vi "_getViDocumentationInfo.vi"(8 "error in (no error)":errorcluster, 11 "VI in":refnum<vi>) -> (0 "error out":errorcluster, 1 "Bookmarks":string[][](array[string]), 2 "VI Documentation Info":T1, 3 "VI out":refnum<vi>)   [LabVIEW 2017]
doc: "Returns the documentation information for the specified VI reference."
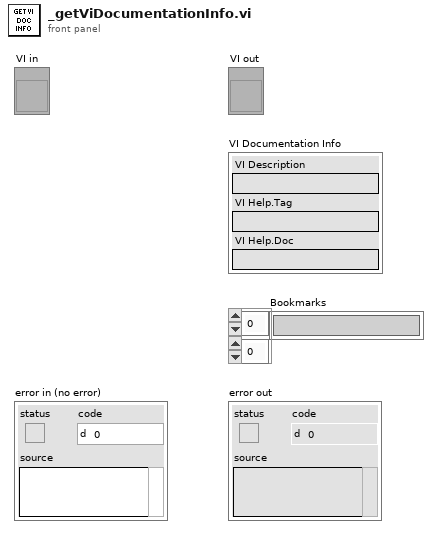
[diagram p1: front panel]
types:
  T1 = cluster{"VI Description":string, "VI Help.Tag":string, "VI Help.Doc":string}
  T2 = cluster{"Description":string, "Help.Tag":string, "Help.URL":string}
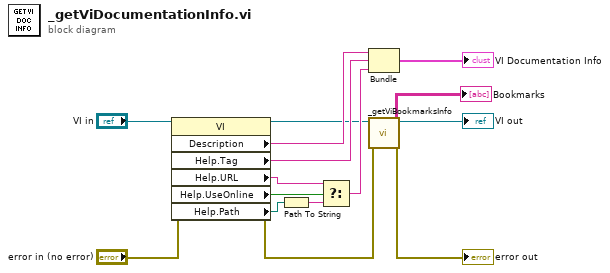
[diagram p0: block diagram]
diagram:
  n1 = property class="VI"(reference="VI in", error in="error in (no error)") -> (reference out=w7:refnum<vi>, error out=w5:errorcluster, "Description"=w13:string, "Help.Tag"=w12:string, "Help.URL"=w3:string, "Help.UseOnline"=w10:bool, "Help.Path"=w11:path)
  n2 = Path To String(path=w11) -> (string=w2:string)
  n3 = Select(t=w3, s=w10, f=w2) -> (s? t:f=w9:string)
  n4 = Bundle("Description"=w13, "Help.Tag"=w12, "Help.URL"=w9) -> (→"VI Documentation Info":T2)  [unwired: 1 in]
  n5 = call "_getViBookmarksInfo.vi"("error in (no error)"=w5, "VI in"=w7) -> ("error out"=→"error out":errorcluster, "Bookmarks"=→"Bookmarks":string[][], "VI out"=→"VI out":refnum<vi>)  [unwired: 7 in]
